vi "Set LakeShore 340 Mode.vi"(4 "enable after power cycle":i32, 5 "units":i32=1, 6 "on/off":i32, 7 "Input chan":string="A", 8 "error in (no error)":errorcluster, 9 "Lake shore mode":T1, 10 "Output #":i32=1, 11 "VISA Resource Name":refnum<visa-resource-name>) -> (0 "error out":errorcluster, 3 "VISA Resource Name Out":refnum<visa-resource-name>)   [LabVIEW 2021]
uses:
  LakeShore340 Mode.ctl
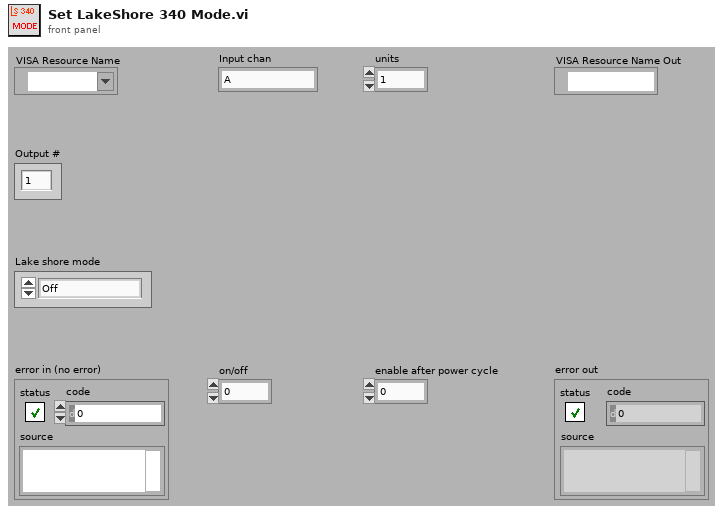
[diagram p1: front panel]
types:
  T1 = typedef "LakeShore340 Mode.ctl" = enum16{"Off", "Manual PID", "Zone", "Open loop", "AutoTune PID", "AutoTune PI", "AutoTune P"}
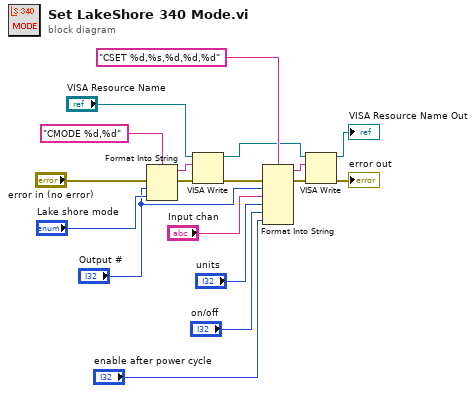
[diagram p0: block diagram]
diagram:
  n1 = Format Into String(format string="CMODE %d,%d" ("data string"), error in="error in (no error)", "Output #", "Lake shore mode") -> (resulting string=w14:string, error out=w16:errorcluster)  [unwired: 1 in]
  n2 = VISA Write(VISA resource name="VISA Resource Name", write buffer=w14, error in (no error)=w16) -> (VISA resource name out=w4:refnum<visa-resource-name>, error out=w2:errorcluster)  [unwired: 1 out]
  n3 = Format Into String(format string="CSET %d,%s,%d,%d,%d" ("data string"), error in=w2, "Output #", "Input chan", "units", "on/off", "enable after power cycle") -> (resulting string=w5:string, error out=w6:errorcluster)  [unwired: 1 in]
  n4 = VISA Write(VISA resource name=w4, write buffer=w5, error in (no error)=w6) -> (VISA resource name out=→"VISA Resource Name Out":refnum<visa-resource-name>, error out=→"error out":errorcluster)  [unwired: 1 out]
